vi "New Wind Turbine.vi"(11 "NXT/EV3":T1) -> ()   [LabVIEW 2016]
uses:
  <vilib>/NXT/Subs/LVHSConnector.ctl
  <vilib>/NXT/LegoClasses/BrickReference/BrickReference.lvclass
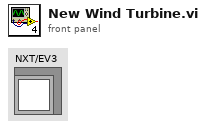
[diagram p1: front panel]
types:
  T1 = typedef "LVHSConnector.ctl" = refnum<class "BrickReference.lvclass">
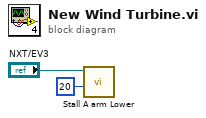
[diagram p0: block diagram]
diagram:
  n1 = call "Stall A arm Lower.vi"("Power"=i8 20, "NXT/EV3"="NXT/EV3") -> ()  [unwired: 9 in, 1 out]
